vi "CalculateValueOfe.vi"() -> ()   [LabVIEW 2018]
panel:
  out "Array":dbl[][](array[numeric])
  out "Numeric":i32
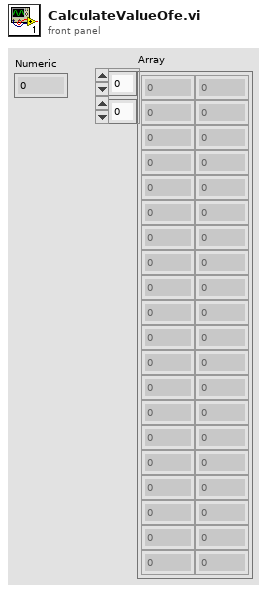
[diagram p1: front panel]
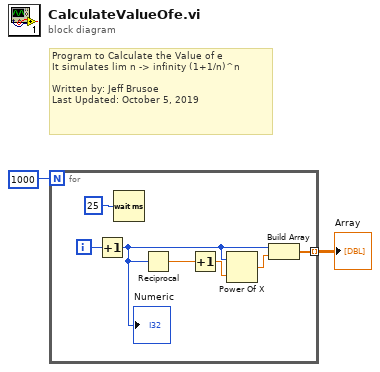
[diagram p0: block diagram]
diagram:
  # "Program to Calculate the Value of e\nIt simulates lim n -> infinity (1+1/n)^n\n\nWritten by: Jeff Brusoe\nLast Updated: October 5, 2019"
  n1 = for {
    N: 1000 -> [_]
    tunnel: [w5] -> w1 mode=indexing
    i -> [w9]
    n2 = Increment(x=w9) -> (x+1=w4:i32)
    "Numeric" <- w4
    n3 = Wait (ms)(milliseconds to wait=u32 25) -> ()  [unwired: 1 out]
    n4 = Reciprocal(x=w4) -> (1/x=w8:dbl)
    n5 = Increment(x=w8) -> (x+1=w7:dbl)
    n6 = Power Of X(1:w7, 2:w4) -> (0:w3:dbl)
    n7 = Build Array(w4, w3) -> (w5:dbl[])
  }
  "Array" <- w1
